vi "Write Name.vi"(8 "error in (no error)":errorcluster, 10 "Name":string, 11 "IViewable In":refnum<class "IViewable.lvclass">) -> (0 "error out":errorcluster, 3 "IViewable Out":refnum<class "IViewable.lvclass">)   [LabVIEW 2015, in "IViewable.lvlib" / "IViewable.lvclass"]
uses:
  IViewable.lvclass
  IViewable.lvclass/IViewable.ctl
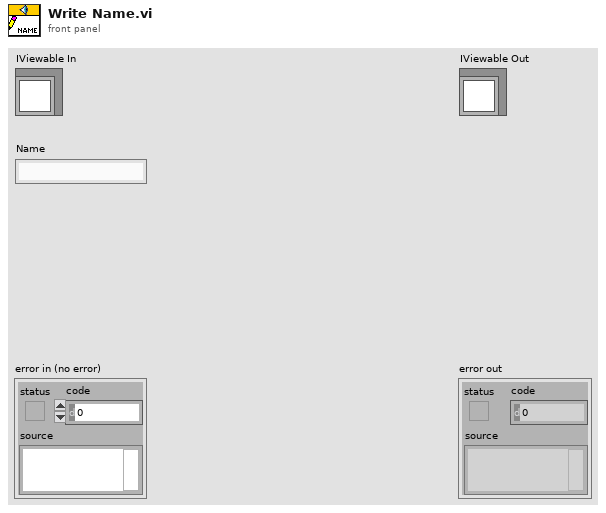
[diagram p1: front panel]
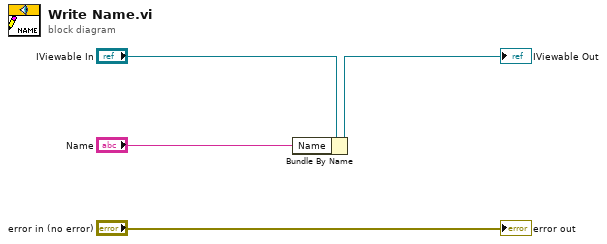
[diagram p0: block diagram]
diagram:
  n1 = Bundle By Name(cluster="IViewable In", "Name"="Name") -> (→"IViewable Out":refnum<class "IViewable.lvclass">)
  "error out" <- "error in (no error)"
